vi "Stop Device.vi"(8 "error in":errorcluster, 11 "Configurable Device in":refnum<class "Configurable Device.lvclass">) -> (0 "error out":errorcluster, 3 "Configurable Device out":refnum<class "Configurable Device.lvclass">)   [LabVIEW 2017, in "Configurable Device.lvclass"]
uses:
  Configurable Device.lvclass
  <vilib>/MSR Consulting, LLC/General Reuse/Session APIs/File Access/Config Data/Config Data.lvclass
  C:/Program Files (x86)/National Instruments/LabVIEW 2017/vi.lib/MSR Consulting, LLC/General Reuse/Session APIs/_Session Fwk/Session - Root.lvclass
  <vilib>/MSR Consulting, LLC/General Reuse/Session APIs/Session Log/System Log.lvclass
  Configurable Device.lvclass/Configurable Device.ctl
  <vilib>/MSR Consulting, LLC/General Reuse/Session APIs/_Session Fwk/Session - Root.lvclass
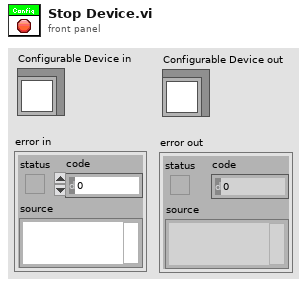
[diagram p1: front panel]
types:
  T1 = typedef "Session - Root.lvclass/Session Handle.ctl" = refnum<data-value>
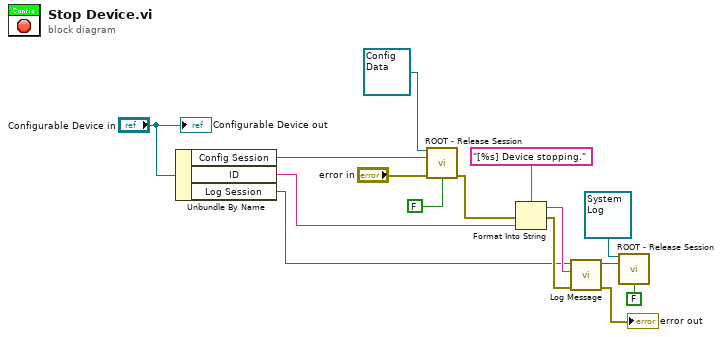
[diagram p0: block diagram]
diagram:
  n1 = Unbundle By Name("Configurable Device in") -> ("Config Session"=w13:T1, "ID"=w9:string, "Log Session"=w1:T1)
  n2 = call <vilib>:"ROOT - Release Session.vi"("OBJ - Session in"=refnum<class "Config Data.lvclass"> refnum ("Config Data"), "Session Handle in"=w13, "error in (no error)"="error in", "force destroy? (F)"=FALSE) -> ("error out"=w8:errorcluster)  [unwired: 10 in, 1 out]
  n3 = Format Into String(format string="[%s] Device stopping.", error in=w8, w9) -> (resulting string=w6:string, error out=w7:errorcluster)  [unwired: 1 in]
  n4 = call <vilib>:"Log Message.vi"("error in"=w7, "MSG In"=w6, "session in"=w1) -> ("error out"=→"error out":errorcluster, "session out"=w5:T1)  [unwired: 7 in]
  n5 = call <vilib>:"ROOT - Release Session.vi"("OBJ - Session in"=refnum<class "System Log.lvclass"> refnum ("Sys Log"), "Session Handle in"=w5, "force destroy? (F)"=FALSE) -> ()  [unwired: 11 in, 2 out]
  "Configurable Device out" <- "Configurable Device in"
